vi "Waveform_Trim (SubVI).vi"(10 "Raw Waveform":ext[][](array[numeric]), 11 "DAQ Sample Window":i32) -> (0 "Second Plane Max Value Index":dbl, 1 "First Plane Max Value Index":dbl, 3 "Trimmed Waveform":ext[][](array[numeric]), 4 "Second Plane":ext[][](graph), 6 "First Plane":ext[][](graph))   [LabVIEW 2013]
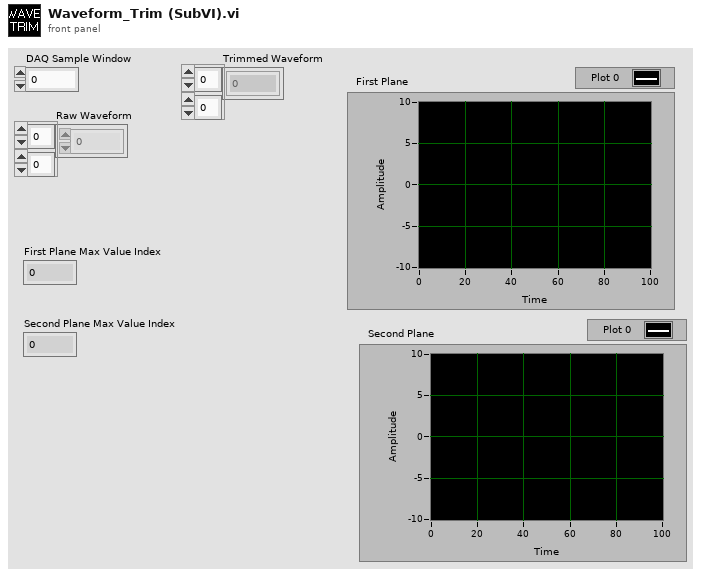
[diagram p1: front panel]
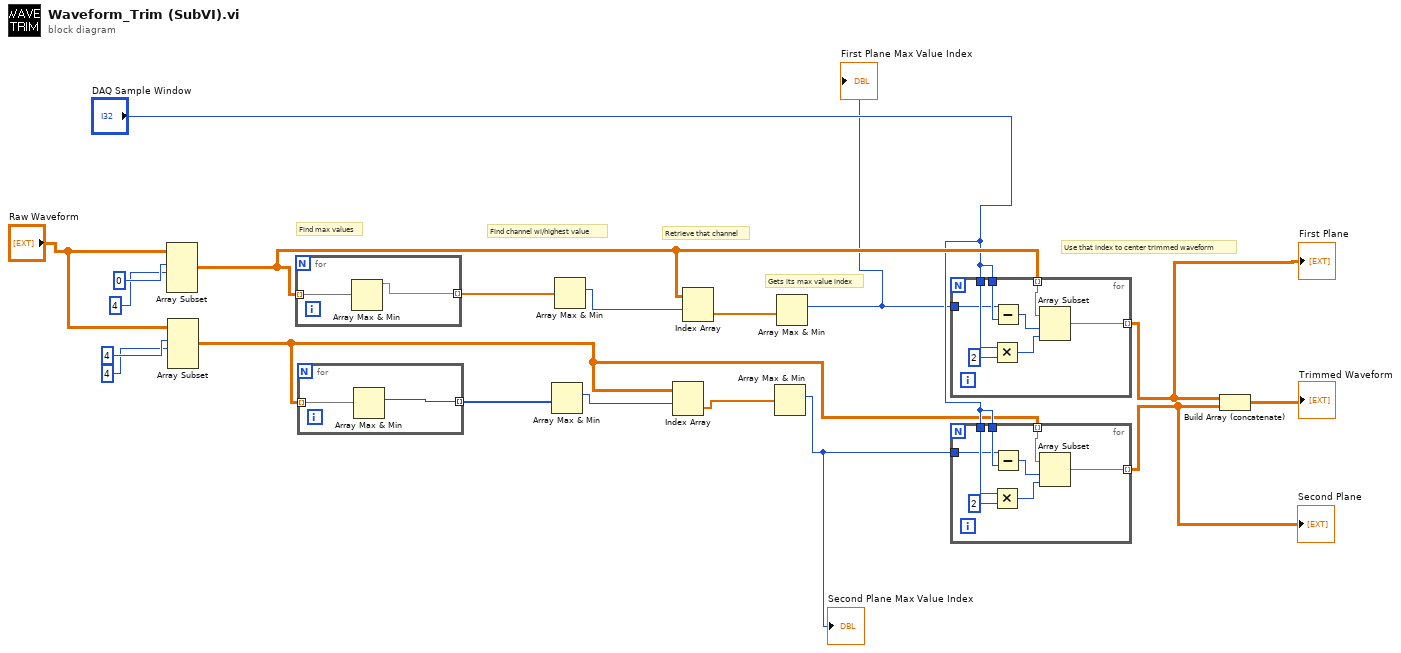
[diagram p0: block diagram]
diagram:
  # "Use that index to center trimmed waveform"
  # "Gets its max value index"
  # "Retrieve that channel"
  # "Find channel wi/highest value"
  # "Find max values"
  n1 = Array Subset(array="Raw Waveform", index (row)=0 ("index"), length (row)=4 ("length")) -> (w15:ext[][])  [unwired: 2 in]
  n2 = Array Subset(array="Raw Waveform", index (row)=4 ("index"), length (row)=4 ("length")) -> (w10:ext[][])  [unwired: 2 in]
  n3 = for {
    tunnel: w15 -> [w21] mode=indexing
    tunnel: [w20] -> w19 mode=indexing
    n4 = Array Max & Min(array=w21) -> (max value=w20:ext)  [unwired: 3 out]
  }
  n5 = for {
    tunnel: w10 -> [w23] mode=indexing
    tunnel: [w22] -> w14 mode=indexing
    n6 = Array Max & Min(array=w23) -> (max index (indices)=w22:i32)  [unwired: 3 out]
  }
  n7 = Array Max & Min(array=w14) -> (max index (indices)=w13:i32)  [unwired: 3 out]
  n8 = Array Max & Min(array=w19) -> (max index (indices)=w17:i32)  [unwired: 3 out]
  n9 = Index Array(array=w10, index (row)=w13) -> (element=w12:ext[])  [unwired: 1 in]
  n10 = Index Array(array=w15, index (row)=w17) -> (element=w16:ext[])  [unwired: 1 in]
  n11 = Array Max & Min(array=w12) -> (max index (indices)=w1:i32)  [unwired: 3 out]
  "Second Plane Max Value Index" <- w1
  n12 = Array Max & Min(array=w16) -> (max index (indices)=w2:i32)  [unwired: 3 out]
  "First Plane Max Value Index" <- w2
  n13 = for {
    tunnel: w15 -> [w29] mode=indexing
    tunnel: "DAQ Sample Window" -> [w31]
    tunnel: "DAQ Sample Window" -> [w27]
    tunnel: [w25] -> w4 mode=indexing
    tunnel: w2 -> [w24]
    n14 = Multiply(x=w27, y=2) -> (x*y=w28:i32)
    n15 = Subtract(x=w24, y=w31) -> (x-y=w30:i32)
    n16 = Array Subset(array=w29, index=w30, length=w28) -> (w25:ext[])
  }
  "First Plane" <- w4
  n17 = for {
    tunnel: w10 -> [w37] mode=indexing
    tunnel: "DAQ Sample Window" -> [w39]
    tunnel: "DAQ Sample Window" -> [w35]
    tunnel: [w33] -> w3 mode=indexing
    tunnel: w1 -> [w32]
    n18 = Multiply(x=w35, y=2) -> (x*y=w36:i32)
    n19 = Subtract(x=w32, y=w39) -> (x-y=w38:i32)
    n20 = Array Subset(array=w37, index=w38, length=w36) -> (w33:ext[])
  }
  "Second Plane" <- w3
  n21 = Build Array (concatenate)(w4, w3) -> (→"Trimmed Waveform":ext[][])
